vi "UtilitySplitCSVStringFromDelimiter.vi"(10 "Delimiter Regular Expression":string, 11 "String in":string) -> (1 "Match Found?":bool, 2 "Before Split":string, 3 "After Split":string)   [LabVIEW 2019, in "flashcards.lvlib"]
uses:
  flashcards.lvlib
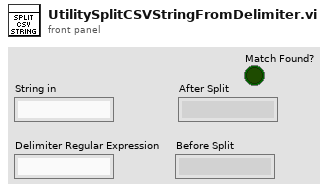
[diagram p1: front panel]
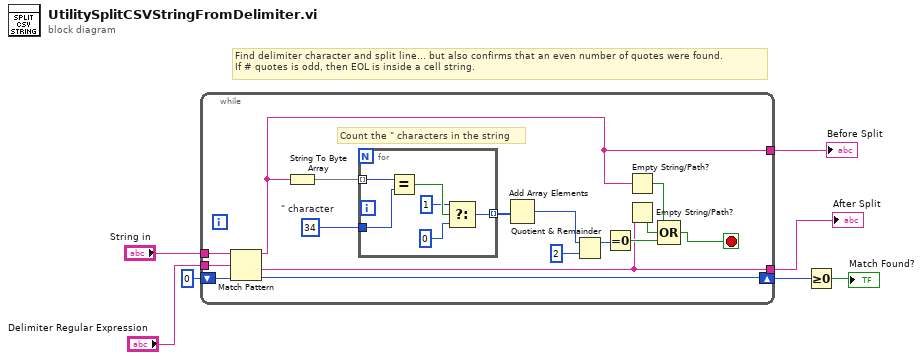
[diagram p0: block diagram]
diagram:
  # "Find delimiter character and split line... but also confirms that an even number of quotes were found.\nIf # quotes is odd, then EOL is inside a cell string."
  n1 = while {
    tunnel: "Delimiter Regular Expression" -> [w23]
    tunnel: [w14] -> w4
    tunnel: "String in" -> [w22]
    tunnel: [w8] -> w6
    shift-right: [w20] -> w2
    shift-left: 0 -> [w21]
    stop <- w16 stop-if-true
    w12 = u8 34  # " character
    # "Count the \" characters in the string"
    n2 = Match Pattern(string=w22, regular expression=w23, offset (0)=w21) -> (before substring=w8:string, after substring=w14:string, offset past match=w20:i32)  [unwired: 1 out]
    n3 = String To Byte Array(string=w8) -> (unsigned byte array=w11:u8[])
    n4 = for {
      tunnel: w12 -> [w29]
      tunnel: w11 -> [w25] mode=indexing
      tunnel: [w24] -> w10 mode=indexing
      n5 = Equal?(x=w25, y=w29) -> (x = y?=w28:bool)
      n6 = Select(t=u8 1, s=w28, f=u8 0 ("length (rest)")) -> (s? t:f=w24:u8)
    }
    n7 = Add Array Elements(numeric array=w10) -> (sum=w9:u8)
    n8 = Quotient & Remainder(x=w9, y=2) -> (x-y*floor(x/y)=w18:i32)  [unwired: 1 out]
    n9 = Equal To 0?(x=w18) -> (x = 0?=w17:bool)
    n10 = Empty String/Path?(string/path=w8) -> (empty?=w13:bool)
    n11 = Empty String/Path?(string/path=w14) -> (empty?=w15:bool)
    n12 = Compound Arithmetic op=OR(w13, w15, w17) -> (w16:bool)
  }
  "Before Split" <- w6
  "After Split" <- w4
  n13 = Greater Or Equal To 0?(x=w2) -> (x >= 0?=→"Match Found?":bool)
